vi "BreakNemaIntoRecordsPerPoint.vi"(7 "elements":string[](array[string]), 8 "IpStatus (in)":T2[](array[typedef]) {"%rtk" scale=0.0..60.0; "TimePing" scale=0.0..60.0}, 11 "IP list":T1) -> (0 "IpStatus (out)":T2[](array[typedef]) {"%rtk" scale=0.0..60.0; "TimePing" scale=0.0..60.0}, 3 "IP list (out)":T1)   [LabVIEW 2011]
uses:
  GPS String Capture Software/IP RTK status Indicator.ctl
  ArrayIpAddressesAndReportingCheckbox.ctl
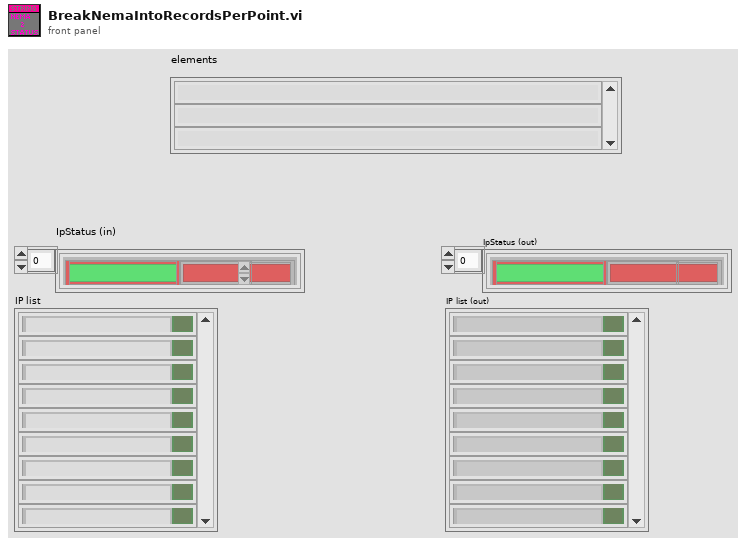
[diagram p1: front panel]
types:
  T1 = typedef "ArrayIpAddressesAndReportingCheckbox.ctl" = cluster{"IpAddress":string, "Report Errors":bool}[]
  T2 = typedef "IP RTK status Indicator.ctl" = cluster{"TimePing":dbl, "IP":string, "%rtk":dbl, "Lastrtk":string, "MinLastRTk":dbl, "RTK Count":bool[], "Last Nema Time":dbl, "Last RTK Time":dbl, "Last Ping time":dbl}
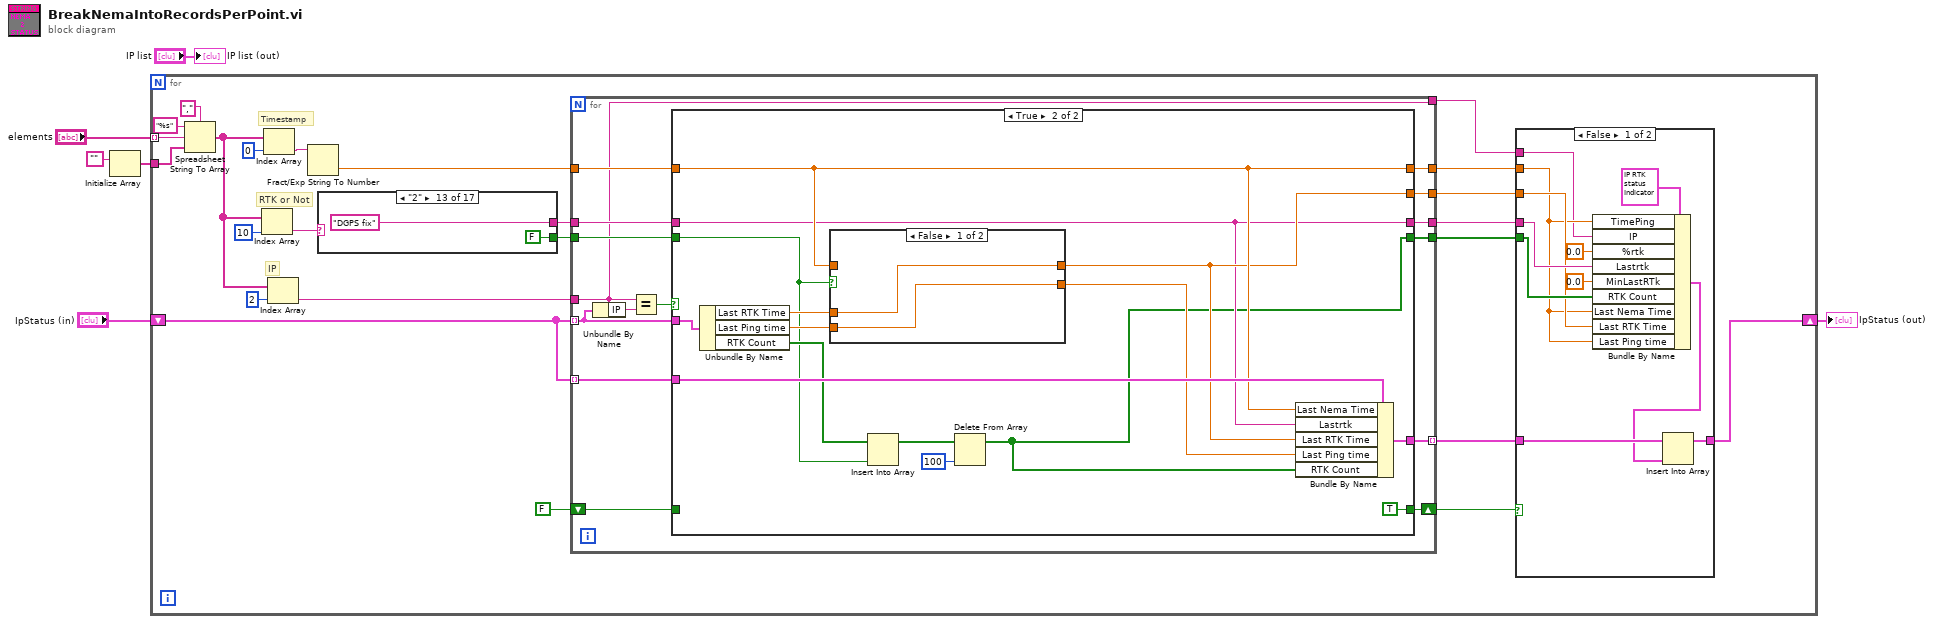
[diagram p0: block diagram]
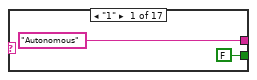
[diagram p3: hidden frame]
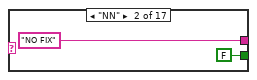
[diagram p4: hidden frame]
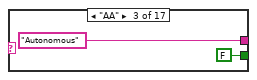
[diagram p5: hidden frame]
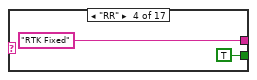
[diagram p6: hidden frame]
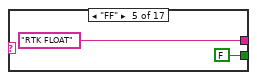
[diagram p7: hidden frame]
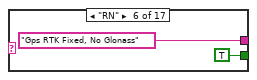
[diagram p8: hidden frame]
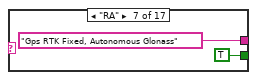
[diagram p9: hidden frame]
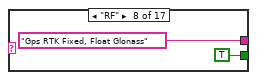
[diagram p10: hidden frame]
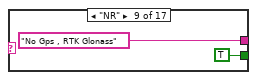
[diagram p11: hidden frame]
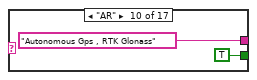
[diagram p12: hidden frame]
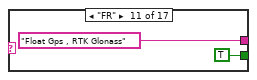
[diagram p13: hidden frame]
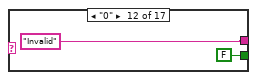
[diagram p14: hidden frame]
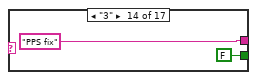
[diagram p15: hidden frame]
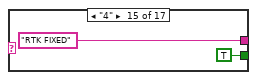
[diagram p16: hidden frame]
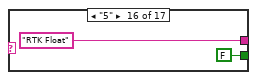
[diagram p17: hidden frame]
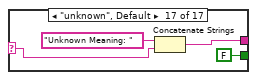
[diagram p18: hidden frame]
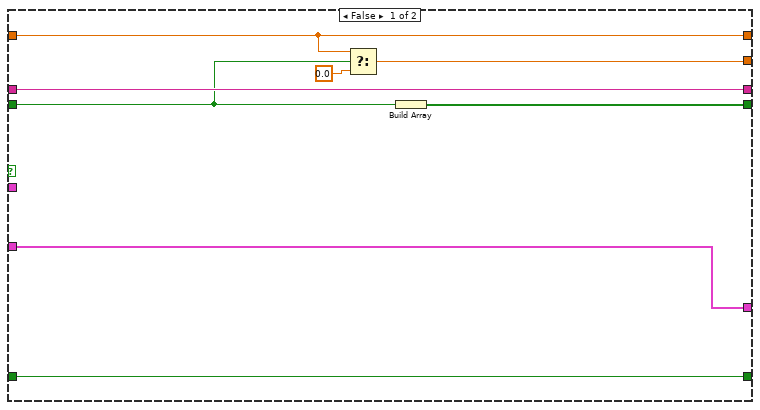
[diagram p19: hidden frame]
diagram:
  n1 = Initialize Array("") -> (w3:string[])  [unwired: 1 in]
  n2 = for {
    tunnel: "elements" -> [w29] mode=indexing
    shift-right: [w14] -> w2
    shift-left: "IpStatus (in)" -> [w17]
    tunnel: w3 -> [w27]
    # "RTK or Not"
    # "IP"
    # "Timestamp"
    n3 = Spreadsheet String To Array(delimiter (Tab)="," ("regular expression"), format string="%s", spreadsheet string=w29, array type (2D Dbl)=w27) -> (array=w21:string[])
    n4 = Index Array(array=w21, index=10) -> (element=w20:string)
    n5 = Index Array(array=w21, index=0) -> (element=w26:string)
    n6 = Index Array(array=w21, index=2) -> (element=w23:string)
    n7 = Fract/Exp String To Number(string=w26) -> (number=w30:dbl)  [unwired: 3 in, 1 out]
    n8 = case shown="\"2\"" w20 {
      selector: w20 -> [_ _ _ _ _ _ _ _ _ _ _ _ _ _ _ _ w76]
      tunnel: ["Autonomous" "NO FIX" "Autonomous" "RTK Fixed" "RTK FLOAT" "Gps RTK Fixed, No Glonass" "Gps RTK Fixed, Autonomous Glonass" "Gps RTK Fixed, Float Glonass" "No Gps , RTK Glonass" "Autonomous Gps , RTK Glonass" "Float Gps , RTK Glonass" "Invalid" "DGPS fix" "PPS fix" "RTK FIXED" "RTK Float" w77] -> w18
      tunnel: [FALSE FALSE FALSE TRUE FALSE TRUE TRUE TRUE TRUE TRUE TRUE FALSE FALSE FALSE TRUE FALSE FALSE] -> w19
      frame "1" {
      }
      frame "NN" {
      }
      frame "AA" {
      }
      frame "RR" {
      }
      frame "FF" {
      }
      frame "RN" {
      }
      frame "RA" {
      }
      frame "RF" {
      }
      frame "NR" {
      }
      frame "AR" {
      }
      frame "FR" {
      }
      frame "0" {
      }
      frame "2" {
      }
      frame "3" {
      }
      frame "4" {
      }
      frame "5" {
      }
      frame "unknown", Default {
        n9 = Concatenate Strings("Unknown Meaning: ", w76) -> (w77:string)
      }
    }
    n10 = for {
      tunnel: w30 -> [w93]
      tunnel: w17 -> [w86] mode=indexing
      tunnel: [w92] -> w13 mode=indexing
      tunnel: w23 -> [w79]
      tunnel: w19 -> [w89]
      tunnel: w18 -> [w88]
      tunnel: w17 -> [w87] mode=indexing
      shift-right: [w84] -> w15
      shift-left: FALSE -> [w85]
      tunnel: [w83] -> w12
      tunnel: [w82] -> w11
      tunnel: [w81] -> w10
      tunnel: [w80] -> w9
      tunnel: [w79] -> w8
      n11 = Unbundle By Name(w86) -> ("IP"=w91:string)
      n12 = Equal?(x=w79, y=w91) -> (x = y?=w90:bool)
      n13 = case shown="True" w90 {
        tunnel: w93 -> [w96 w105]
        tunnel: [w101 w116] -> w92
        tunnel: w89 -> [w97 w109]
        tunnel: w88 -> [w99 w103]
        tunnel: w87 -> [w101 w115]
        tunnel: w86 -> [_ w114]
        tunnel: w85 -> [w100 _]
        tunnel: [w100 TRUE] -> w84
        tunnel: [w96 w105] -> w83
        tunnel: [w99 w103] -> w82
        tunnel: [w98 w102] -> w81
        tunnel: [w94 w104] -> w80
        frame False {
          n14 = Select(t=w96, s=w97, f=0.0) -> (s? t:f=w94:dbl)
          n15 = Build Array(w97) -> (w98:bool[])
        }
        frame True {
          n16 = Unbundle By Name(w114) -> ("Last RTK Time"=w113:dbl, "Last Ping time"=w111:dbl, "RTK Count"=w110:bool[])
          n17 = case shown="False" w109 {
            tunnel: w113 -> [w118 _]
            tunnel: w105 -> [_ w119]
            tunnel: [w118 w119] -> w104
            tunnel: [w117 w119] -> w112
            tunnel: w111 -> [w117 _]
            frame False {
            }
            frame True {
            }
          }
          n18 = Insert Into Array(array=w110, new element=w109) -> (w108:bool[])  [unwired: 1 in]
          n19 = Delete From Array(array=w108, index=100) -> (array with subset deleted=w102:bool[])  [unwired: 1 in, 1 out]
          n20 = Bundle By Name(cluster=w115, "Last Nema Time"=w105, "Lastrtk"=w103, "Last RTK Time"=w104, "Last Ping time"=w112, "RTK Count"=w102) -> (w116:T2)
        }
      }
    }
    n21 = case shown="False" w15 {
      tunnel: [w40 w42] -> w14
      tunnel: w13 -> [w41 w42]
      tunnel: w12 -> [w34 _]
      tunnel: w11 -> [w37 _]
      tunnel: w10 -> [w36 _]
      tunnel: w9 -> [w35 _]
      tunnel: w8 -> [w33 _]
      frame False {
        n22 = Bundle By Name(cluster=T2 {"TimePing"=0.0, "IP"="", "%rtk"=0.0, "Lastrtk"="", "MinLastRTk"=0.0, "RTK Count"=[], "Last Nema Time"=0.0, "Last RTK Time"=0.0, "Last Ping time"=0.0} ("IP Status"), "TimePing"=w34, "IP"=w33, "%rtk"=0.0, "Lastrtk"=w37, "MinLastRTk"=0.0, "RTK Count"=w36, "Last Nema Time"=w34, "Last RTK Time"=w35, "Last Ping time"=w34) -> (w38:T2)
        n23 = Insert Into Array(array=w41, new element=w38) -> (w40:T2[])  [unwired: 1 in]
      }
      frame True {
      }
    }
  }
  "IpStatus (out)" <- w2
  "IP list (out)" <- "IP list"
